vi "05Foot.vi"() -> ()   [LabVIEW 2015]
uses:
  <vilib>/Utility/error.llb/DialogType.ctl
  <vilib>/Instr/_visa.llb/VISA Configure Serial Port (Serial Instr).vi
  <vilib>/Utility/file.llb/Read Delimited Spreadsheet (DBL).vi
panel:
  in  "Tab Control":T1(tab)
  out "INC":dbl min=0.0 max=12.0 step=0.1 format="%.1g"
  out "MPH":dbl min=0.0 max=12.0 step=0.1 format="%.1g"
  out "Error":string
  out "Time ms Start":u32
  out "Index":i32
  out "Dwell":dbl[](array[numeric])
  out "Time":dbl[](array[numeric])
  out "Speed":dbl[](array[numeric])
  in  "Command":string
  in  "Insert Command":bool
  out "Part":string
  in  "Port":refnum<visa-resource-name>="COM8"
  out "Data":T2
  out "FootMsg":string
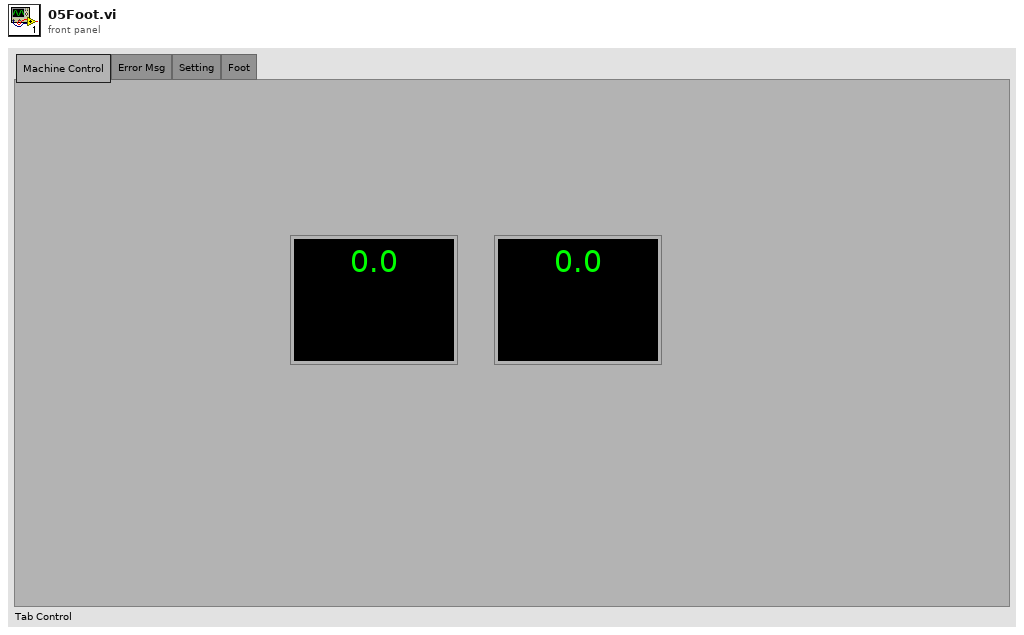
[diagram p1: front panel]
types:
  T1 = enum32{"Machine Control", "Error Msg", "Setting", "Foot"}
  T2 = cluster{"err":i32[], "vin":i32, "vbus":i32, "amps":i32, "iamp":i32, "mph":i32, "inc":i32}
  T3 = enum16{"Initialize", "Close", "Next", "Send", "GetScript", "GetMPH", "NextMPH"}
  T4 = enum32{"Machine Control", "Error Msg", "Setting"}
  T5 = enum16{"Initialize", "Close", "Next", "Send", "GetScript"}
  T6 = enum16{"Initialize", "FootReceive", "FootDisplay"}
  T7 = enum16{"Initialize", "Next", "Send RSET", "Set MPH", "Set INC", "Part to 0", "Get MPH"}
  T8 = enum16{"Initialize", "Next", "Send RSET", "Set MPH", "Set INC", "Part to 0"}
  T9 = enum16{"Initialize", "Close", "Next", "Send", "GetScript", "GetMPH"}
  T10 = typedef "DialogType.ctl" = u16
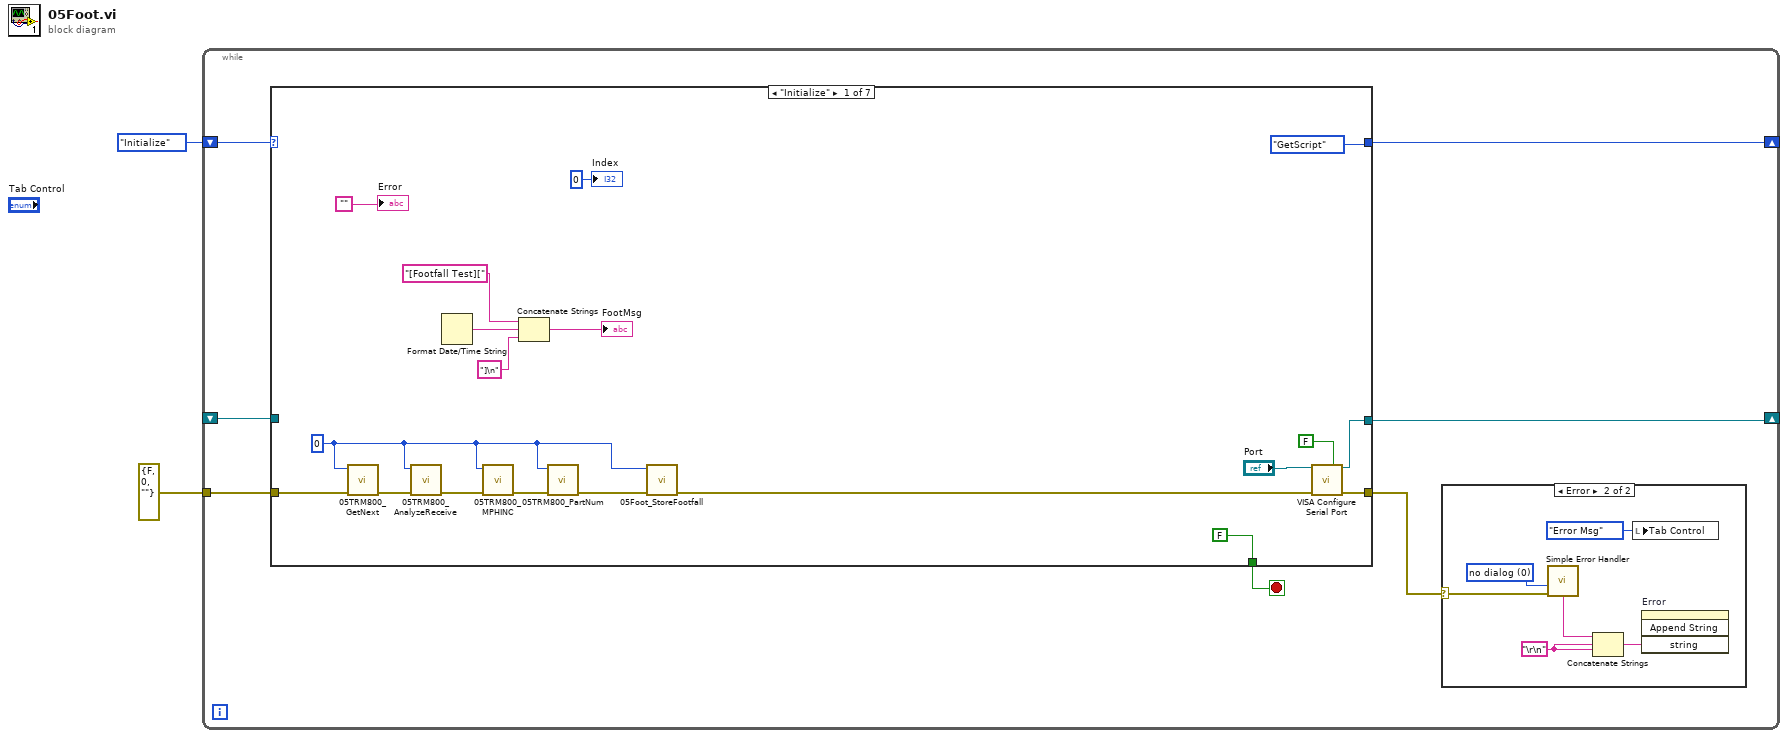
[diagram p0: block diagram]
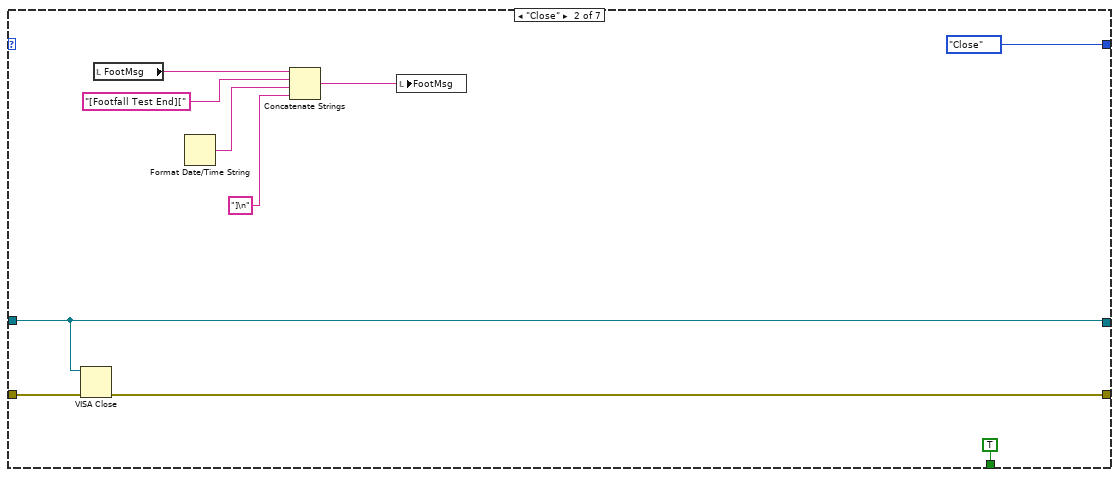
[diagram p3: hidden frame]
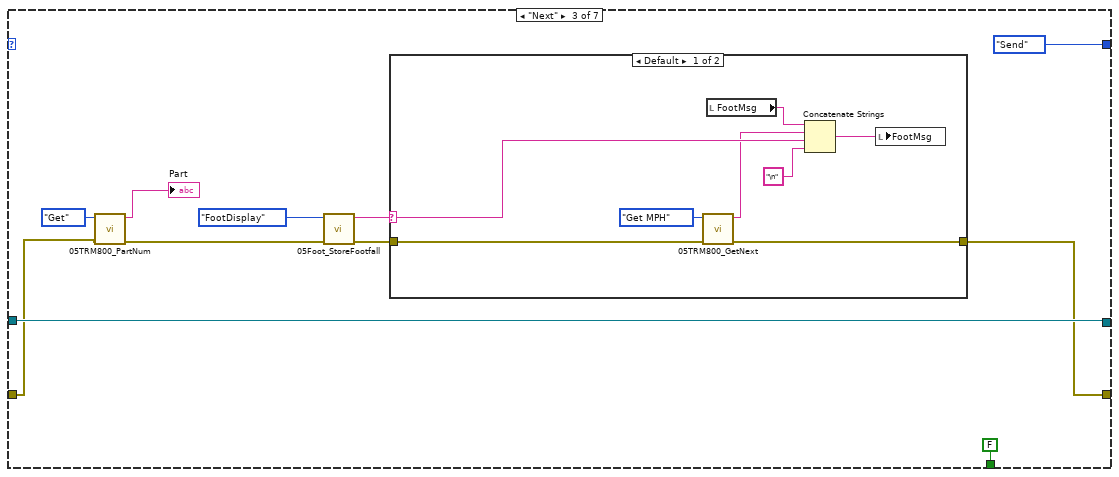
[diagram p4: hidden frame]
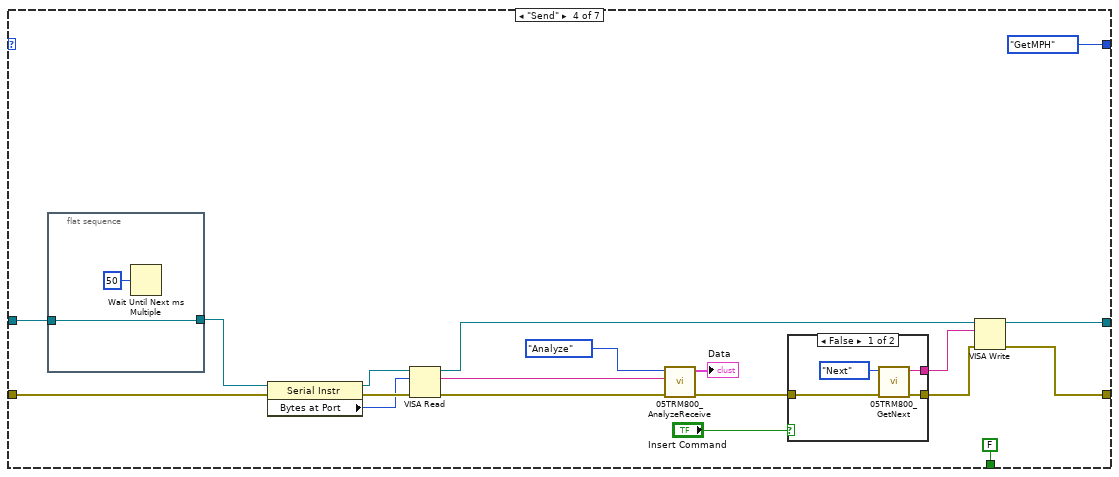
[diagram p6: hidden frame]
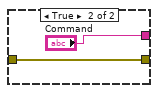
[diagram p7: hidden frame]
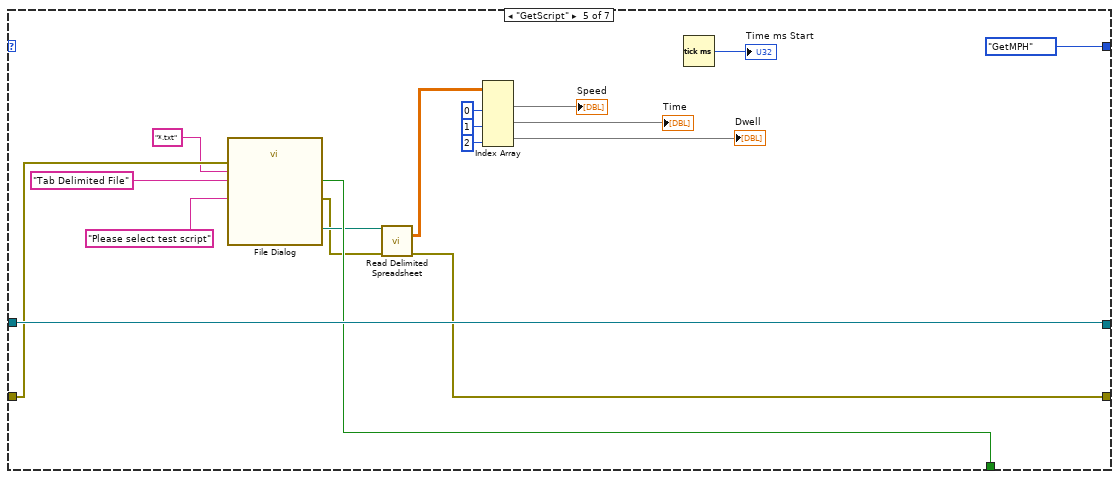
[diagram p8: hidden frame]
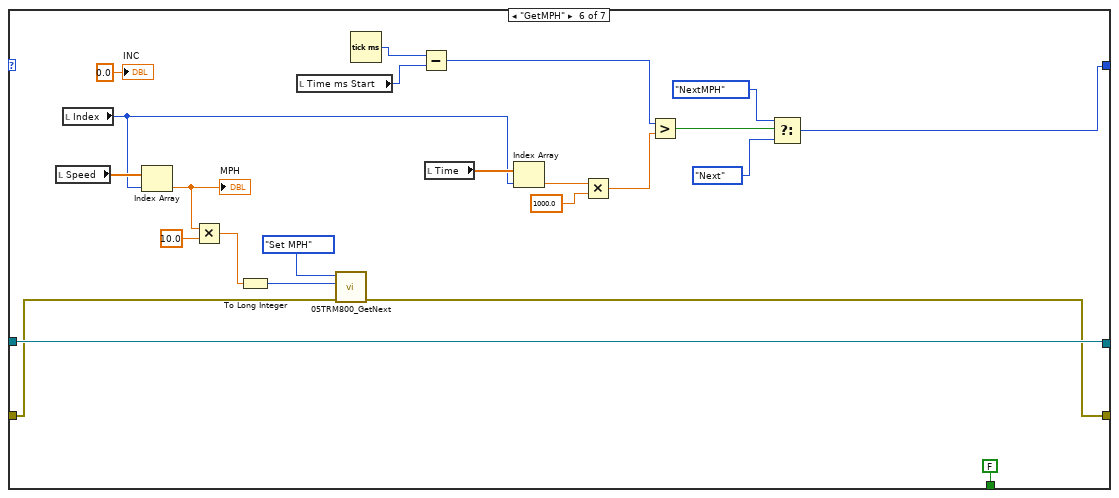
[diagram p9: hidden frame]
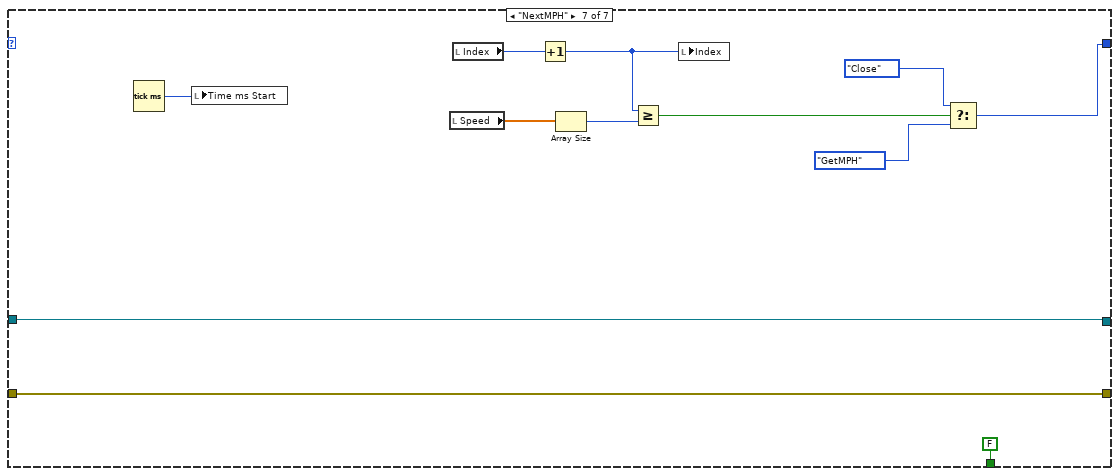
[diagram p10: hidden frame]
diagram:
  n1 = while {
    shift-right: [w8] -> _
    shift-left: T3."Initialize" -> [w9]
    tunnel: errorcluster {"status"=FALSE, "code"=0, "source"=""} ("error constant") -> [w6]
    shift-right: [w4] -> _
    shift-left: _ -> [w3]
    stop <- w7 stop-if-true
    n2 = case shown="\"Initialize\"" w9 {
      tunnel: [T5."GetScript" enum16{"Initialize", "Close"}."Close" T3."Send" T3."GetMPH" T9."GetMPH" w112 w134] -> w8
      tunnel: [FALSE TRUE FALSE FALSE w106 FALSE ("cancelled") FALSE ("cancelled")] -> w7
      tunnel: w6 -> [w29 w42 w46 w81 w108 w130 w143]
      tunnel: [w33 w40 w48 w75 w102 w129 w143] -> w5
      tunnel: [w30 w41 w54 w76 w109 w132 w142] -> w4
      tunnel: w3 -> [_ w41 w54 w83 w109 w132 w142]
      frame "Initialize" {
        w25 = u16 0
        n3 = call "05TRM800_GetNext.vi"("error in (no error)"=w29, "Enum"=w25) -> ("error out"=w28:errorcluster)  [unwired: 8 in, 1 out]
        n4 = call "05TRM800_AnalyzeReceive.vi"("error in (no error)"=w28, "Enum"=w25) -> ("error out"=w27:errorcluster)  [unwired: 8 in, 1 out]
        n5 = Format Date/Time String() -> (date/time string=w17:string)  [unwired: 3 in]
        n6 = call "05TRM800_MPHINC.vi"("error in (no error)"=w27, "Enum"=w25) -> ("error out"=w26:errorcluster)  [unwired: 7 in, 2 out]
        n7 = Concatenate Strings("[Footfall Test][", w17, "]\n") -> (→"FootMsg":string)
        n8 = call "05TRM800_PartNum.vi"("error in (no error)"=w26, "Enum"=w25) -> ("error out"=w24:errorcluster)  [unwired: 8 in, 1 out]
        n9 = call "05Foot_StoreFootfall.vi"("error in (no error)"=w24, "Enum"=w25) -> ("error out"=w23:errorcluster)  [unwired: 8 in, 1 out]
        n10 = call-poly "VISA Configure Serial Port"("VISA resource name"="Port", "Enable Termination\nChar (T)"=FALSE ("Enable Termination\nChar (T)"), "error in (no error)"=w23) -> ("VISA resource name out"=w30:refnum<visa-resource-name>, "error out"=w33:errorcluster)  [unwired: 11 in]
        "Error" <- ""
        "Index" <- 0 ("Index")
      }
      frame "Close" {
        n11 = VISA Close(VISA resource name=w41, error in (no error)=w42) -> (error out=w40:errorcluster)
        n12 = local read "FootMsg"() -> (w39:string)
        n13 = Format Date/Time String() -> (date/time string=w37:string)  [unwired: 3 in]
        n14 = Concatenate Strings(w39, "[Footfall Test End][" ("string"), w37, "]\n") -> (w35:string)
        n15 = local write "FootMsg"(w35) -> ()
      }
      frame "Next" {
        n16 = call "05TRM800_PartNum.vi"("error in (no error)"=w46, "Enum"=enum16{"Initialize", "Get", "Input"}."Get") -> ("error out"=w51:errorcluster, "Part Num"=→"Part":string)  [unwired: 8 in]
        n17 = call "05Foot_StoreFootfall.vi"("error in (no error)"=w51, "Enum"=T6."FootDisplay") -> ("error out"=w47:errorcluster, "FootOut"=w49:string)  [unwired: 8 in]
        n18 = case shown="Default" w49 {
          selector: w49 -> [w60 _]
          tunnel: [w58 w64] -> w48
          tunnel: w47 -> [w57 w64]
          frame Default {
            n19 = call "05TRM800_GetNext.vi"("error in (no error)"=w57, "Enum"=T7."Get MPH") -> ("error out"=w58:errorcluster, "String"=w59:string)  [unwired: 8 in]
            n20 = local read "FootMsg"() -> (w63:string)
            n21 = Concatenate Strings(w63, w59, w60, "\n" ("string")) -> (w62:string)
            n22 = local write "FootMsg"(w62) -> ()
          }
          frame "" {
          }
        }
      }
      frame "Send" {
        n23 = flat-sequence {
          tunnel: w83 -> [w90]
          tunnel: [w90] -> w82
          frame #0 {
            n24 = Wait Until Next ms Multiple(millisecond multiple=u32 50) -> ()  [unwired: 1 out]
          }
        }
        n25 = property class="Serial Instr"(reference=w82, error in=w81) -> (reference out=w79:refnum<visa-resource-name>, error out=w80:errorcluster, "Bytes at Port"=w78:u32)
        n26 = VISA Read(VISA resource name=w79, byte count=w78, error in (no error)=w80) -> (VISA resource name out=w77:refnum<visa-resource-name>, read buffer=w70:string, error out=w65:errorcluster)  [unwired: 1 out]
        n27 = call "05TRM800_AnalyzeReceive.vi"("error in (no error)"=w65, "String"=w70, "Enum"=enum16{"Initialize", "Analyze"}."Analyze") -> ("error out"=w71:errorcluster, "Data"=→"Data":T2)  [unwired: 7 in]
        n28 = case shown="False" "Insert Command" {
          tunnel: [w87 "Command"] -> w73
          tunnel: [w86 w88] -> w72
          tunnel: w71 -> [w85 w88]
          frame False {
            n29 = call "05TRM800_GetNext.vi"("error in (no error)"=w85, "Enum"=T8."Next") -> ("error out"=w86:errorcluster, "String"=w87:string)  [unwired: 8 in]
          }
          frame True {
          }
        }
        n30 = VISA Write(VISA resource name=w77, write buffer=w73, error in (no error)=w72) -> (VISA resource name out=w76:refnum<visa-resource-name>, error out=w75:errorcluster)  [unwired: 1 out]
      }
      frame "GetScript" {
        n31 = call "File Dialog"("prompt"="Please select test script", "error in"=w108, "pattern (all files)"="*.txt", "pattern label"="Tab Delimited File") -> ("selected path"=w104:path, "cancelled"=w106:bool, "error out"=w103:errorcluster)  [unwired: 8 in, 1 out]
        n32 = call-poly <vilib>:"Read Delimited Spreadsheet.vi"("file path (dialog if empty)"=w104, "error in (no error)"=w103) -> ("all rows"=w97:dbl[][], "error out"=w102:errorcluster)  [unwired: 8 in, 4 out]
        n33 = Index Array(array=w97, index (col) #1=0 ("disabled index (col)"), index (col) #2=1 ("index (col)"), index (col) #3=2 ("index (col)")) -> (element #1=→"Speed":dbl[], element #2=→"Time":dbl[], element #3=→"Dwell":dbl[])  [unwired: 3 in]
        n34 = Tick Count (ms)() -> (millisecond timer value=→"Time ms Start":u32)
      }
      frame "GetMPH" {
        n35 = local read "Speed"() -> (w126:dbl[])
        n36 = local read "Index"() -> (w120:i32)
        n37 = Index Array(array=w126, index=w120) -> (element=w125:dbl)
        "MPH" <- w125
        n38 = Multiply(x=w125, y=10.0) -> (x*y=w111:dbl)
        n39 = To Long Integer(number=w111) -> (32bit integer=w110:i32)
        n40 = local read "Time ms Start"() -> (w122:u32)
        n41 = call "05TRM800_GetNext.vi"("error in (no error)"=w130, "Value"=w110, "Enum"=T8."Set MPH") -> ("error out"=w129:errorcluster)  [unwired: 7 in, 1 out]
        n42 = Tick Count (ms)() -> (millisecond timer value=w123:u32)
        n43 = Subtract(x=w123, y=w122) -> (x-y=w117:u32)
        n44 = local read "Time"() -> (w121:dbl[])
        n45 = Index Array(array=w121, index=w120) -> (element=w119:dbl)
        n46 = Multiply(x=w119, y=1000.0) -> (x*y=w116:dbl)
        n47 = Greater?(x=w117, y=w116) -> (0:w115:bool)
        n48 = Select(t=T3."NextMPH", s=w115, f=T3."Next") -> (s? t:f=w112:T3)
        "INC" <- 0.0 ("INC")
      }
      frame "NextMPH" {
        n49 = Tick Count (ms)() -> (millisecond timer value=w133:u32)
        n50 = local write "Time ms Start"(w133) -> ()
        n51 = local read "Speed"() -> (w140:dbl[])
        n52 = local read "Index"() -> (w141:i32)
        n53 = Increment(x=w141) -> (x+1=w139:i32)
        n54 = Array Size(array=w140) -> (size(s)=w138:i32)
        n55 = Greater Or Equal?(x=w139, y=w138) -> (x >= y?=w136:bool)
        n56 = local write "Index"(w139) -> ()
        n57 = Select(t=T3."Close", s=w136, f=T3."GetMPH") -> (s? t:f=w134:T3)
      }
    }
    n58 = case shown="Error" w5 {
      selector: w5 -> [_ w14]
      frame No Error {
      }
      frame Error {
        w11 = "\r\n"
        w15 = T10 0 items=["no dialog", "OK message", "continue or stop message", "OK message + warnings", "continue/stop + warnings"] ("type of dialog (OK msg:1)")
        n59 = call <vilib>:"Simple Error Handler.vi"("type of dialog (OK msg:1)"=w15, "error in (no error)"=w14) -> ("message"=w12:string)  [unwired: 3 in, 4 out]
        n60 = Concatenate Strings(w12, w11, w11) -> (w13:string)
        n61 = local write "Tab Control"(T4."Error Msg" ("Tab Control")) -> ()
        n62 = invoke on="Error" class="Str" method="Append String"("string"=w13) -> ()  [unwired: 3 in, 4 out]
      }
    }
  }
